vi "Configure OVP Level.vi"(8 "error in":errorcluster, 9 "Level(V)":dbl min=0.0 format="%.2g", 11 "VISA resource name":refnum<visa-resource-name>) -> (0 "error out":errorcluster, 3 "VISA resource name out":refnum<visa-resource-name>)   [LabVIEW 2015, in "IT6700H.lvlib"]
doc: "This command is used to set the upper voltage limit of the OVP for overvoltage protection. If the peak output voltage is higher than the OVP upper limit, the output of the power supply is shorted internally and the \"OV\" bit of the query status register is set. After the overvoltage protection state occurs, you can send the VOLT:PROT:CLE command to clear the overvoltage protection state.\n<b>Level(V)</b>\n0-MAX"
uses:
  <instrlib>/IT6700H/IT6700H.lvlib
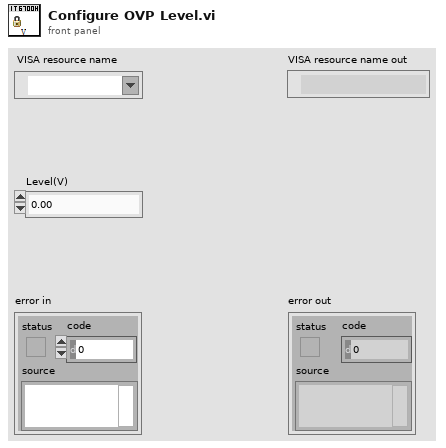
[diagram p1: front panel]
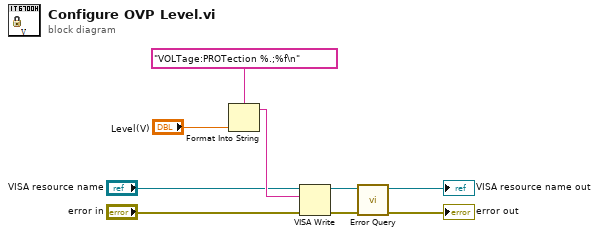
[diagram p0: block diagram]
diagram:
  n1 = Format Into String(format string="VOLTage:PROTection %.;%f\n", "Level(V)") -> (resulting string=w7:string)  [unwired: 2 in, 1 out]
  n2 = VISA Write(VISA resource name="VISA resource name", write buffer=w7, error in (no error)="error in") -> (VISA resource name out=w3:refnum<visa-resource-name>, error out=w4:errorcluster)  [unwired: 1 out]
  n3 = call <instrlib>:"Error Query.vi"("error in"=w4, "VISA resource name"=w3) -> ("error out"=→"error out":errorcluster, "VISA resource name out"=→"VISA resource name out":refnum<visa-resource-name>)  [unwired: 6 in, 2 out]
